vi "GetFlatSequenceFrameReference.vi"(8 "error in":errorcluster, 11 "FlatSequence in":refnum<class "FlatSequenceFrame.lvclass">) -> (0 "error out":errorcluster, 1 "reference out":refnum<vi>, 3 "FlatSequence out":refnum<class "FlatSequenceFrame.lvclass">)   [LabVIEW 2014, in "FlatSequenceFrame.lvclass"]
uses:
  FlatSequenceFrame.lvclass
  Generic/Generic.lvclass
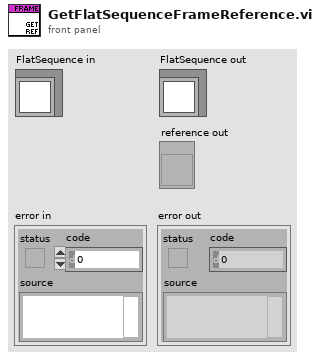
[diagram p1: front panel]
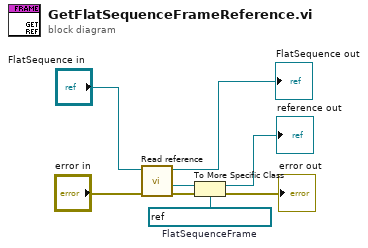
[diagram p0: block diagram]
diagram:
  w8 = refnum<vi> refnum  # FlatSequenceFrame
  n1 = call "Read reference.vi"("error in"="error in", "GObject in"="FlatSequence in") -> ("error out"=w7:errorcluster, "reference"=w6:refnum<vi>, "GObject out"=→"FlatSequence out":refnum<class "FlatSequenceFrame.lvclass">)  [unwired: 5 in]
  n2 = To More Specific Class(target class=w8, reference=w6, error in=w7) -> (specific class reference=→"reference out":refnum<vi>, error out=→"error out":errorcluster)
